vi "Drive Core.vi"   [LabVIEW 2014]
uses:
  <vilib>/Rock Robotics/WPI/DriverStation/WPI_DriverStationRobotMode2.ctl
  Begin/Global Variables.vi
  Begin/Global Constants.vi
types:
  T1 = typedef "WPI_DriverStationRobotMode2.ctl" = enum16{"Autonomous Disabled", "Autonomous Enabled", "Teleop Disabled", "Teleop Enabled", "Disconnected", "Finish", "Test Disabled", "Test Enabled", "Emergency Stopped"}
  T2 = cluster{"Header P":dbl, "Header I":dbl, "Header D":dbl}
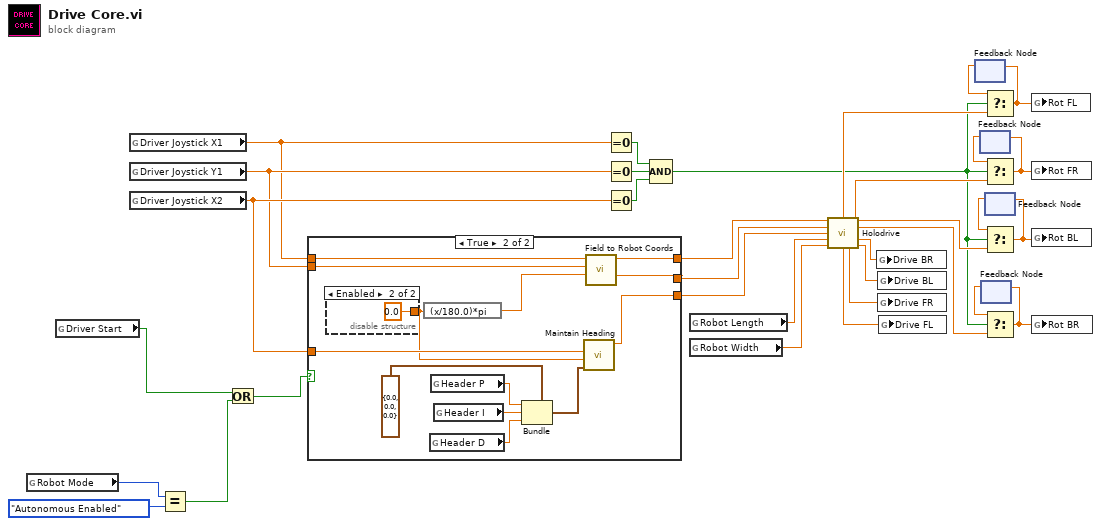
[diagram p0: block diagram]
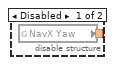
[diagram p3: hidden frame]
diagram:
  n1 = global read "Global Variables.vi" "Robot Mode"() -> (w29:T1)
  n2 = global read "Global Variables.vi" "Driver Start"() -> (w1:bool)
  n3 = global read "Global Variables.vi" "Driver Joystick X1"() -> (w25:dbl)
  n4 = global read "Global Variables.vi" "Driver Joystick Y1"() -> (w26:dbl)
  n5 = global read "Global Variables.vi" "Driver Joystick X2"() -> (w30:dbl)
  n6 = Equal?(x=w29, y=WPI_DriverStationRobotMode2."Autonomous Enabled") -> (x = y?=w3:bool)
  n7 = Or(x=w1, y=w3) -> (x .or. y?=w2:bool)
  n8 = case shown="True" w2 {
    tunnel: w25 -> [w36 w49]
    tunnel: w26 -> [w35 w48]
    tunnel: [w36 w47] -> w27
    tunnel: [w35 w46] -> w28
    tunnel: w30 -> [w34 w45]
    tunnel: [w34 w44] -> w31
    frame False {
    }
    frame True {
      n9 = disable-structure shown="Enabled" {
        disable-tunnel: [w50 0.0 ("NavX Yaw")] -> w37
        frame Disabled {
          n10 = global read "Global Variables.vi" "NavX Yaw"() -> (w50:dbl)
        }
        frame Enabled {
        }
      }
      n11 = expression code="(x/180.0)*pi" ("degrees to radians")(w37) -> (w43:dbl)
      n12 = global read "Global Constants.vi" "Header D"() -> (w40:dbl)
      n13 = global read "Global Constants.vi" "Header P"() -> (w42:dbl)
      n14 = global read "Global Constants.vi" "Header I"() -> (w41:dbl)
      n15 = Bundle(cluster=T2 {"Header P"=0.0, "Header I"=0.0, "Header D"=0.0}, "Header P"=w42, "Header I"=w41, "Header D"=w40) -> (w39:T2)
      n16 = call "Maintain Heading.vi"("PID gains"=w39, "NavX Yaw"=w37, "Raw Driver Joystick X2"=w45) -> ("Driver Joystick X2"=w44:dbl)  [unwired: 8 in]
      n17 = call "Field to Robot Coords.vi"("gyro"=w43, "Joystick y"=w48, "Joystick x"=w49) -> ("robot y"=w46:dbl, "robot x"=w47:dbl)  [unwired: 7 in]
    }
  }
  n18 = Equal To 0?(x=w25) -> (x = 0?=w8:bool)
  n19 = Equal To 0?(x=w26) -> (x = 0?=w9:bool)
  n20 = Equal To 0?(x=w30) -> (x = 0?=w10:bool)
  n21 = Compound Arithmetic op=AND(w8, w9, w10) -> (w11:bool)
  n22 = global read "Global Constants.vi" "Robot Length"() -> (w32:dbl)
  n23 = global read "Global Constants.vi" "Robot Width"() -> (w33:dbl)
  n24 = call "Holodrive.vi"("Translation X"=w27, "Translation Y"=w28, "Angular"=w31, "Robot Length"=w32, "Robot Width"=w33) -> ("FL Rot"=w17:dbl, "FR Rot"=w14:dbl, "BL Rot"=w15:dbl, "BR Rot"=w16:dbl, "BR Drive"=w7:dbl, "FL Drive"=w4:dbl, "FR Drive"=w5:dbl, "BL Drive"=w6:dbl)  [unwired: 3 in]
  n25 = global write "Global Variables.vi" "Drive BR"(w7) -> ()
  n26 = global write "Global Variables.vi" "Drive BL"(w6) -> ()
  n27 = global write "Global Variables.vi" "Drive FR"(w5) -> ()
  n28 = global write "Global Variables.vi" "Drive FL"(w4) -> ()
  n29 = feedback #1() -> (w19:dbl)  [unwired: 1 in]
  n30 = feedback #2() -> (w13:dbl)  [unwired: 1 in]
  n31 = feedback #3() -> (w23:dbl)  [unwired: 1 in]
  n32 = Select(t=w19, s=w11, f=w17) -> (s? t:f=w18:dbl)
  n33 = feedback-in #1(w18) -> ()
  n34 = Select(t=w13, s=w11, f=w14) -> (s? t:f=w12:dbl)
  n35 = feedback-in #2(w12) -> ()
  n36 = feedback #4() -> (w21:dbl)  [unwired: 1 in]
  n37 = Select(t=w21, s=w11, f=w15) -> (s? t:f=w20:dbl)
  n38 = feedback-in #4(w20) -> ()
  n39 = Select(t=w23, s=w11, f=w16) -> (s? t:f=w22:dbl)
  n40 = feedback-in #3(w22) -> ()
  n41 = global write "Global Variables.vi" "Rot FL"(w18) -> ()
  n42 = global write "Global Variables.vi" "Rot FR"(w12) -> ()
  n43 = global write "Global Variables.vi" "Rot BL"(w20) -> ()
  n44 = global write "Global Variables.vi" "Rot BR"(w22) -> ()
